vi "Pause.vi"(8 "error in (no error)":errorcluster, 11 "Timer in":refnum<class "Timer.lvclass">) -> (0 "error out":errorcluster, 3 "Timer out":refnum<class "Timer.lvclass">)   [LabVIEW 2020, in "Timer.lvclass"]
uses:
  Timer.lvclass
  Timer.lvclass/Timer.ctl
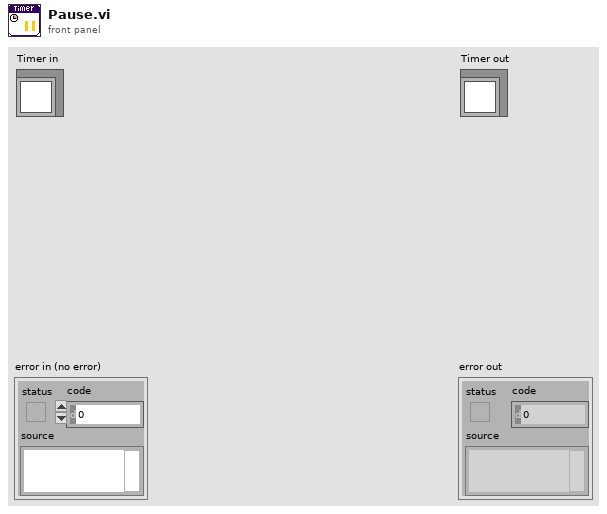
[diagram p1: front panel]
types:
  T1 = cluster{"target time(ms)":u32, "elapsed time(ms)":u32, "start time":u32, "pause":bool, "auto reset":bool}
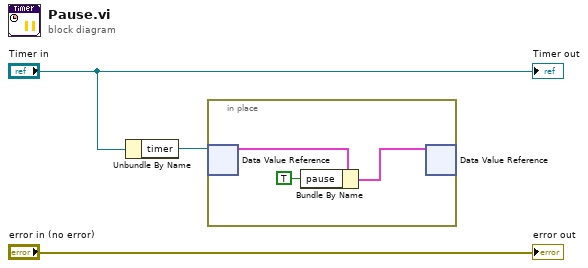
[diagram p0: block diagram]
diagram:
  n1 = Unbundle By Name("Timer in") -> ("timer"=w1:refnum<data-value>)
  n2 = in-place {
    n3 = in-place-dvr #1(w1) -> (w6:T1)  [unwired: 1 out]
    n4 = Bundle By Name(cluster=w6, "pause"=TRUE) -> (w4:T1)
    n5 = in-place-dvr #1(w4) -> ()  [unwired: 2 out]
  }
  "error out" <- "error in (no error)"
  "Timer out" <- "Timer in"
